vi "System Explorer - Add PPL content to System Explorer library.vi"(6 "Support Runtime Configuration":bool, 8 "error in (no error)":errorcluster, 9 "Extra Page Names":string[](array[string]), 10 "Project Root":path, 11 "CD Wizard - Internal Data":T1) -> (0 "error out":errorcluster, 2 "VIs to Process":path[](array[path]), 3 "subVIs to replace":path[](array[path]))   [LabVIEW 2020, in "NIVS_Consolidated_CDW_MetaDataObj.lvclass"]
doc: "Add all virtual folders and VIs to the System Explorer library."
uses:
  NIVS_Consolidated_CDW_MetaDataObj.lvclass
  Internal data.ctl
  CD System Explorer lvlib.ctl
  Add Item - Type.ctl
  CD System Explorer lvlib.vi
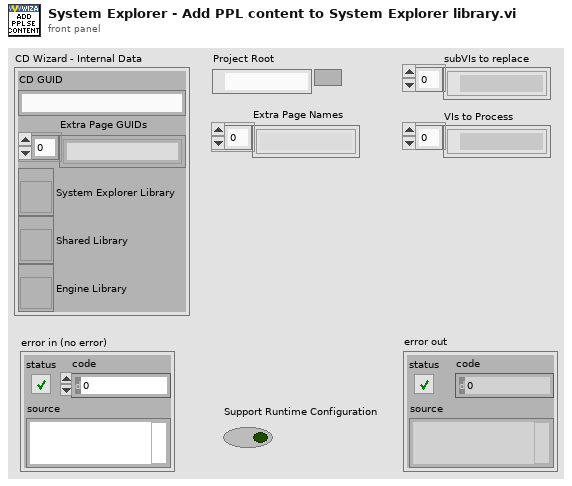
[diagram p1: front panel]
types:
  T1 = typedef "NIVS_Consolidated_CDW_MetaDataObj.lvclass/Internal data.ctl" = cluster{"CD GUID":string, "Extra Page GUIDs":string[], "System Explorer Library":refnum<vi>, "Shared Library":refnum<vi>, "Engine Library":refnum<vi>}
  T2 = typedef "NIVS_Consolidated_CDW_MetaDataObj.lvclass/CD System Explorer lvlib.ctl" = enum16{"LibraryFileName", "LibraryFolderName", "System Explorer.FolderName", "System Explorer.Dynamically Called.FolderName", "System Explorer.Dynamically Called.Extra Pages.FolderName", "System Explorer.Dynamically Called.Extra Pages.TemplatePathAndName", "System Explorer.Dynamically Called.Main Page.VIName", "System Explorer.Dynamically Called.Main Page.TemplatePathAndName", "System Explorer.Dynamically Called.Initialization VI.VIName", "System Explorer.Dynamically Called.Initialization VI.TemplatePathAndName", "System Explorer.SubVI.FolderName", "System Explorer.Types.FolderName", "System Explorer.ActionVIOnCompile.VIName", "System Explorer.ActionVIOnRecompile.VIName", "System Explorer.ExportConfigRTM.VIName", "System Explorer.PPL.ExportConfigRTM.VIName", "System Explorer.LoadHelpFile.VIName", "System Explorer.PPL.LoadHelpFile.VIName", "System Explorer.SetRTDriverVIsFilePaths.VIName", "System Explorer.ClearRTDriverVIs.VIName"}
  T3 = typedef "NIVS_Consolidated_CDW_MetaDataObj.lvclass/Add Item - Type.ctl" = string
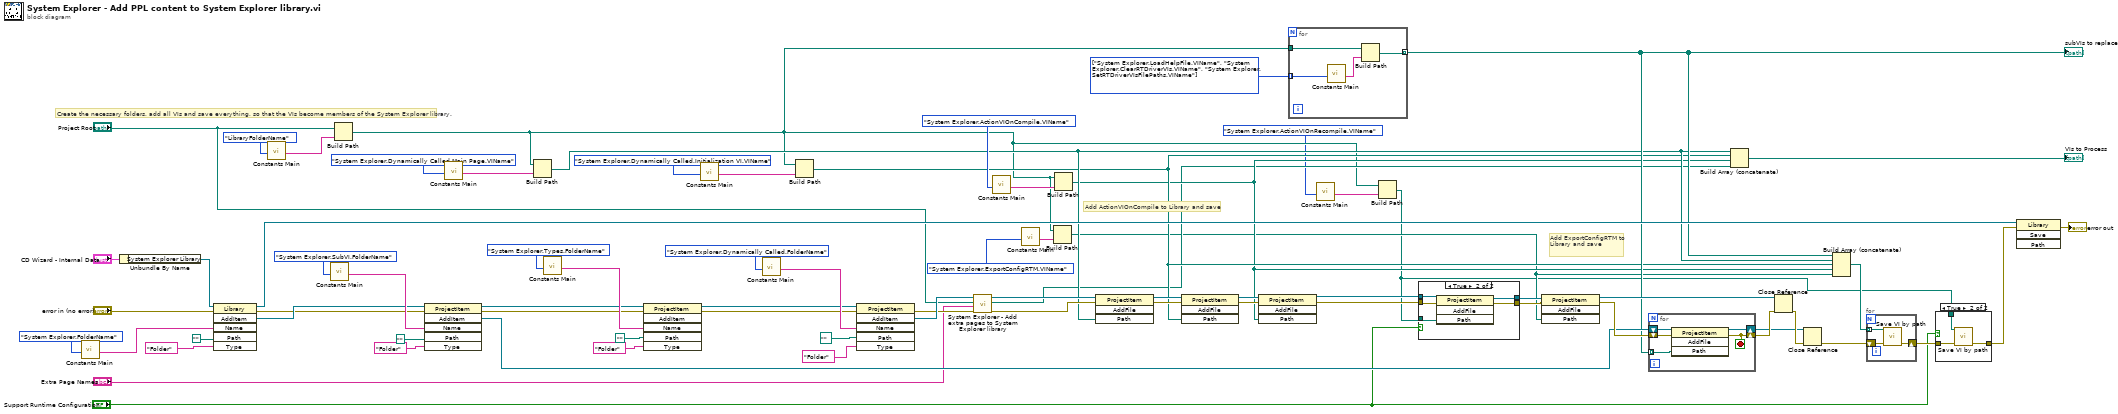
[diagram p0: block diagram]
diagram:
  w21 = T2[] [enum."System Explorer.LoadHelpFile.VIName", enum."System Explorer.ClearRTDriverVIs.VIName", enum."System Explorer.SetRTDriverVIsFilePaths.VIName"] items=["LibraryFileName", "LibraryFolderName", "System Explorer.FolderName", "System Explorer.Dynamically Called.FolderName", "System Explorer.Dynamically Called.Extra Pages.FolderName", "System Explorer.Dynamically Called.Extra Pages.TemplatePathAndName", "System Explorer.Dynamically Called.Main Page.VIName", "System Explorer.Dynamically Called.Main Page.TemplatePathAndName", "System Explorer.Dynamically Called.Initialization VI.VIName", "System Explorer.Dynamically Called.Initialization VI.TemplatePathAndName", "System Explorer.SubVI.FolderName", "System Explorer.Types.FolderName", "System Explorer.ActionVIOnCompile.VIName", "System Explorer.ActionVIOnRecompile.VIName", "System Explorer.ExportConfigRTM.VIName", "System Explorer.PPL.ExportConfigRTM.VIName", "System Explorer.LoadHelpFile.VIName", "System Explorer.PPL.LoadHelpFile.VIName", "System Explorer.SetRTDriverVIsFilePaths.VIName", "System Explorer.ClearRTDriverVIs.VIName"]
  # "Create the necessary folders, add all VIs and save everything, so that the VIs become members of the System Explorer library."
  # "Add ExportConfigRTM to Library and save"
  # "Add ActionVIOnCompile to Library and save"
  n1 = call-poly "Constants Main.vi"("Action"=CD_System_Explorer_lvlib."System Explorer.FolderName") -> ("Output"=w69:string)  [unwired: 10 in]
  n2 = Unbundle By Name("CD Wizard - Internal Data") -> ("System Explorer Library"=w46:refnum<vi>)
  n3 = invoke class="Library" method="AddItem"(reference=w46, error in="error in (no error)", "Name"=w69, "Path"=path "", "Type"=T3 "Folder" ("Add Item - Type")) -> (reference out=w48:refnum<vi>, error out=w27:errorcluster, "AddItem"=w47:refnum<vi>)  [unwired: 1 in, 3 out]
  n4 = call-poly "Constants Main.vi"("Action"=CD_System_Explorer_lvlib."LibraryFolderName") -> ("Output"=w41:string)  [unwired: 10 in]
  n5 = call-poly "Constants Main.vi"("Action"=CD_System_Explorer_lvlib."System Explorer.SubVI.FolderName") -> ("Output"=w63:string)  [unwired: 10 in]
  n6 = Build Path(base path="Project Root", name or relative path=w41) -> (appended path=w11:path)
  n7 = invoke class="ProjectItem" method="AddItem"(reference=w47, error in=w27, "Name"=w63, "Path"=path "", "Type"=T3 "Folder" ("Add Item - Type")) -> (reference out=w50:refnum<vi>, error out=w26:errorcluster, "AddItem"=w29:refnum<vi>)  [unwired: 1 in, 3 out]
  n8 = call-poly "Constants Main.vi"("Action"=CD_System_Explorer_lvlib."System Explorer.Dynamically Called.Main Page.VIName") -> ("Output"=w67:string)  [unwired: 10 in]
  n9 = Build Path(base path=w11, name or relative path=w67) -> (appended path=w17:path)
  n10 = call-poly "Constants Main.vi"("Action"=CD_System_Explorer_lvlib."System Explorer.Types.FolderName") -> ("Output"=w58:string)  [unwired: 10 in]
  n11 = invoke class="ProjectItem" method="AddItem"(reference=w50, error in=w26, "Name"=w58, "Path"=path "", "Type"=T3 "Folder" ("Add Item - Type")) -> (reference out=w49:refnum<vi>, error out=w25:errorcluster)  [unwired: 1 in, 4 out]
  n12 = call-poly "Constants Main.vi"("Action"=CD_System_Explorer_lvlib."System Explorer.Dynamically Called.Initialization VI.VIName") -> ("Output"=w66:string)  [unwired: 10 in]
  n13 = call-poly "Constants Main.vi"("Action"=CD_System_Explorer_lvlib."System Explorer.Dynamically Called.FolderName") -> ("Output"=w53:string)  [unwired: 10 in]
  n14 = Build Path(base path=w11, name or relative path=w66) -> (appended path=w16:path)
  n15 = invoke class="ProjectItem" method="AddItem"(reference=w49, error in=w25, "Name"=w53, "Path"=path "", "Type"=T3 "Folder" ("Add Item - Type")) -> (error out=w43:errorcluster, "AddItem"=w45:refnum<vi>)  [unwired: 1 in, 4 out]
  n16 = call "System Explorer - Add extra pages to System Explorer library.vi"("error in (no error)"=w43, "Extra Page Names"="Extra Page Names", "Project Root"="Project Root", "ProjectItem in"=w45) -> ("error out"=w24:errorcluster, "Extra Page VIs"=w13:path[], "ProjectItem out"=w44:refnum<vi>)  [unwired: 5 in]
  n17 = call-poly "Constants Main.vi"("Action"=CD_System_Explorer_lvlib."System Explorer.ActionVIOnCompile.VIName") -> ("Output"=w37:string)  [unwired: 10 in]
  n18 = call-poly "Constants Main.vi"("Action"=CD_System_Explorer_lvlib."System Explorer.ExportConfigRTM.VIName") -> ("Output"=w33:string)  [unwired: 10 in]
  n19 = Build Path(base path=w11, name or relative path=w33) -> (appended path=w5:path)
  n20 = Build Path(base path=w11, name or relative path=w37) -> (appended path=w15:path)
  n21 = invoke class="ProjectItem" method="AddFile"(reference=w44, error in=w24, "Path"=w17) -> (reference out=w51:refnum<vi>, error out=w52:errorcluster)  [unwired: 1 in, 2 out]
  n22 = invoke class="ProjectItem" method="AddFile"(reference=w51, error in=w52, "Path"=w16) -> (reference out=w40:refnum<vi>, error out=w39:errorcluster)  [unwired: 1 in, 2 out]
  n23 = invoke class="ProjectItem" method="AddFile"(reference=w40, error in=w39, "Path"=w15) -> (reference out=w9:refnum<vi>, error out=w7:errorcluster)  [unwired: 1 in, 2 out]
  n24 = for {
    tunnel: w21 -> [w78] mode=indexing
    tunnel: w11 -> [w76]
    tunnel: [w75] -> w18 mode=indexing
    n25 = call-poly "Constants Main.vi"("Action"=w78) -> ("Output"=w77:string)  [unwired: 10 in]
    n26 = Build Path(base path=w76, name or relative path=w77) -> (appended path=w75:path)
  }
  "subVIs to replace" <- w18
  n27 = call-poly "Constants Main.vi"("Action"=CD_System_Explorer_lvlib."System Explorer.ActionVIOnRecompile.VIName") -> ("Output"=w12:string)  [unwired: 10 in]
  n28 = Build Path(base path=w11, name or relative path=w12) -> (appended path=w1:path)
  n29 = case shown="True" "Support Runtime Configuration" {
    tunnel: w9 -> [w80 w85]
    tunnel: [w80 w84] -> w8
    tunnel: w7 -> [w79 w83]
    tunnel: [w79 w82] -> w6
    tunnel: w1 -> [_ w81]
    frame False {
    }
    frame True {
      n30 = invoke class="ProjectItem" method="AddFile"(reference=w85, error in=w83, "Path"=w81) -> (reference out=w84:refnum<vi>, error out=w82:errorcluster)  [unwired: 1 in, 2 out]
    }
  }
  n31 = invoke class="ProjectItem" method="AddFile"(reference=w8, error in=w6, "Path"=w5) -> (reference out=w31:refnum<vi>, error out=w36:errorcluster)  [unwired: 1 in, 2 out]
  n32 = for {
    shift-right: [w86] -> w32
    shift-left: w36 -> [w90]
    shift-right: [w89] -> w30
    shift-left: w29 -> [w88]
    tunnel: w18 -> [w87] mode=indexing
    stop <- w86 stop-if-true
    n33 = invoke class="ProjectItem" method="AddFile"(reference=w88, error in=w90, "Path"=w87) -> (reference out=w89:refnum<vi>, error out=w86:errorcluster)  [unwired: 1 in, 2 out]
  }
  n34 = Build Array (concatenate)(w17, w16, w15, w13) -> (→"VIs to Process":path[])
  n35 = Close Reference(reference=w31, error in (no error)=w32) -> (error out=w35:errorcluster)
  n36 = Close Reference(reference=w30, error in (no error)=w35) -> (error out=w19:errorcluster)
  n37 = Build Array (concatenate)(w18, w17, w16, w15, w5) -> (w20:path[])
  n38 = for {
    tunnel: w20 -> [w93] mode=indexing
    shift-right: [w91] -> w4
    shift-left: w19 -> [w92]
    n39 = call "Save VI by path.vi"("error in (no error)"=w92, "VI path"=w93) -> ("error out"=w91:errorcluster)  [unwired: 9 in]
  }
  n40 = case shown="True" "Support Runtime Configuration" {
    tunnel: w4 -> [w94 w97]
    tunnel: [w94 w96] -> w3
    tunnel: w1 -> [_ w95]
    frame False {
    }
    frame True {
      n41 = call "Save VI by path.vi"("error in (no error)"=w97, "VI path"=w95) -> ("error out"=w96:errorcluster)  [unwired: 9 in]
    }
  }
  n42 = invoke class="Library" method="Save"(reference=w48, error in=w3) -> (error out=→"error out":errorcluster)  [unwired: 2 in, 3 out]
